vi "ChangeState.vi"(6 "interface object in":refnum<k20>, 8 "error in (no error)":errorcluster, 10 "state":u16(ring)=128 items=["start remote node"=1, "stop remote node"=2, "enter pre-operational"=128, "reset node"=129, "reset communication"=130], 11 "MotorControllerClass in":refnum<class "MotorControllerClass.lvclass">) -> (0 "error out":errorcluster, 1 "interface object out":refnum<k20>, 3 "MotorControllerClass out":refnum<class "MotorControllerClass.lvclass">)   [LabVIEW 2018, in "MotorControllerClass.lvclass"]
uses:
  BMS/MotorControllerClass.lvclass
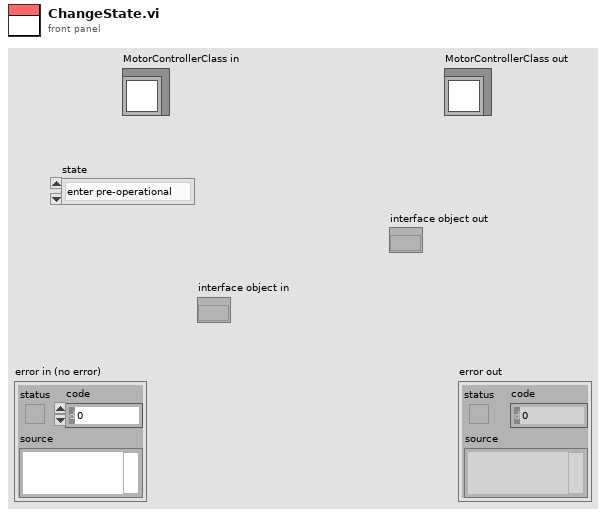
[diagram p1: front panel]
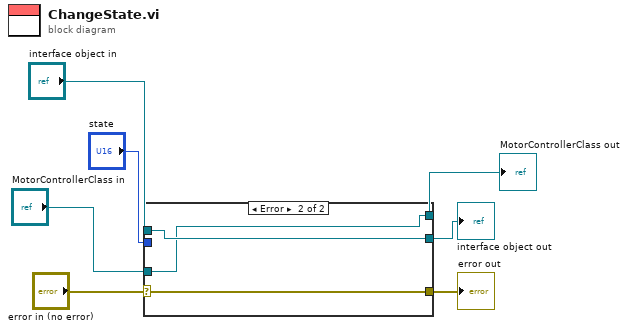
[diagram p0: block diagram]
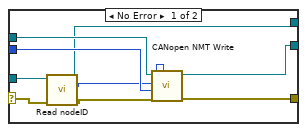
[diagram p2: hidden frame]
diagram:
  n1 = case shown="Error" "error in (no error)" {
    selector: "error in (no error)" -> [w10 w19]
    tunnel: [w13 w19] -> w6
    tunnel: "state" -> [w16 _]
    tunnel: "interface object in" -> [w15 w18]
    tunnel: [w14 w18] -> w3
    tunnel: "MotorControllerClass in" -> [w9 w17]
    tunnel: [w8 w17] -> w1
    frame No Error {
      n2 = call-dynamic "Read nodeID.vi"("error in (no error)"=w10, "MotorControllerClass in"=w9) -> ("error out"=w11:errorcluster, "nodeID"=w12:u8, "MotorControllerClass out"=w8:refnum<class "MotorControllerClass.lvclass">)  [unwired: 7 in]
      n3 = call <vilib>:"CANopen NMT Write.vi"("node-ID (0)"=w12, "error in (no error)"=w11, "command"=w16, "interface object in"=w15) -> ("error out"=w13:errorcluster, "interface object out"=w14:refnum<k20>)  [unwired: 6 in]
    }
    frame Error {
    }
  }
  "error out" <- w6
  "interface object out" <- w3
  "MotorControllerClass out" <- w1
